vi "Start Sequence.vi"(8 "error in (no error)":errorcluster, 11 "SequencingModel in":refnum<class "SequencingModel.lvclass">) -> (0 "error out":errorcluster, 3 "SequencingModel out":refnum<class "SequencingModel.lvclass">)   [LabVIEW 2017, in "SequencingModel.lvlib" / "SequencingModel.lvclass"]
uses:
  <vilib>/gpm_packages/@cs/example/Dynamic Viewables/SequencingModel/SequencingModel.lvclass
  <vilib>/gpm_packages/@cs/example/Dynamic Viewables/SequencingModel/SequencingModel.lvclass/SequencingModel.ctl
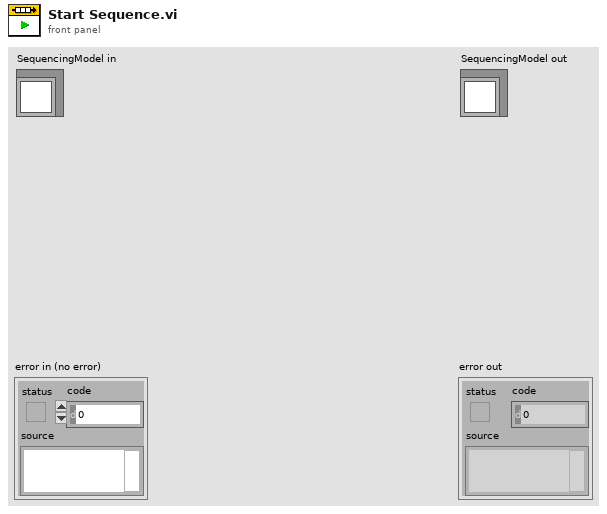
[diagram p1: front panel]
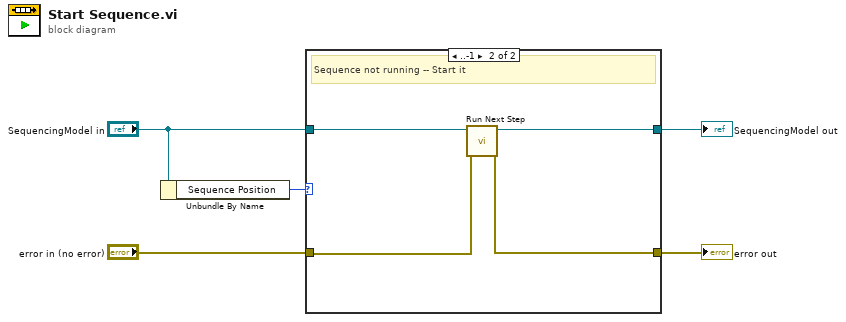
[diagram p0: block diagram]
diagram:
  n1 = Unbundle By Name("SequencingModel in") -> ("Sequence Position"=w1:i32)
  n2 = case shown="..-1" w1 {
    tunnel: "error in (no error)" -> [w6 w9]
    tunnel: "SequencingModel in" -> [w7 w11]
    tunnel: [w6 w8] -> w4
    tunnel: [w7 w10] -> w3
    frame 0.. {
      # "Sequence is running -- Ignore start"
    }
    frame ..-1 {
      # "Sequence not running -- Start it"
      n3 = call <vilib>:"Run Next Step.vi"("error in (no error)"=w9, "SequencingModel in"=w11) -> ("error out"=w8:errorcluster, "SequencingModel out"=w10:refnum<class "SequencingModel.lvclass">)  [unwired: 8 in]
    }
  }
  "error out" <- w4
  "SequencingModel out" <- w3
